vi "ziExample-PWA_SignalInput.vi"() -> ()   [LabVIEW 2009]
doc: "Control a Zurich instrument device via the LabOne Labview API. \nRequirements: Zurich Instruments UHFLI \nThis example retrives Periodic Waveform Analyzer (PWA) data from an UHFLI instrument.\n\n© Zurich Instruments AG, www.zhinst.com\\"
uses:
  <instrlib>/Zurich Instruments LabOne/Public/Data/ziTypePWAWave.ctl
  <instrlib>/Zurich Instruments LabOne/Public/Configure/ziSetValueDoubleArray.vi
  <vilib>/Analysis/2dsp.llb/Real FFT.vi
  <instrlib>/Zurich Instruments LabOne/Public/Data/ziGetEventPWAWave.vi
  <instrlib>/Zurich Instruments LabOne/Zurich Instruments LabOne.lvlib
  <vilib>/Analysis/NI_AALPro.lvlib
  <vilib>/Analysis/NI_AALBase.lvlib
panel:
  out "Error Out":errorcluster
  out "Selected Device":string
  in  "Address":string="DEV"
  in  "Bins":i32=512
  in  "stop":bool
  out "PWAWave":T1={"Timestamp (ticks)"=2149, "SampleCount"=0, "InputSelect"=0, "OscSelect"=0, "Harmonic"=0, "BinCount"=0, "Frequency (Hz)"=0.0, "PWAType"=0, "Mode"=0, "Overflow"=0, "Commensurable"=0, "BinPhase"=[], "X"=[], "Y"=[], "countBin"=[]} {"Frequency (Hz)" format="%#_6p"}
  out "FFT / Harmonics":dbl[](graph)
  out "Waveform":cluster{dbl[], dbl[]}(graph)
  out "Counts per Bin":cluster{dbl[], u32[]}(graph)
  # "ziExample-PWA.vi\nRequirements: UHFLI\nsee block diagram for VI description"
  # "Tested Devices:\n- UHFLI"
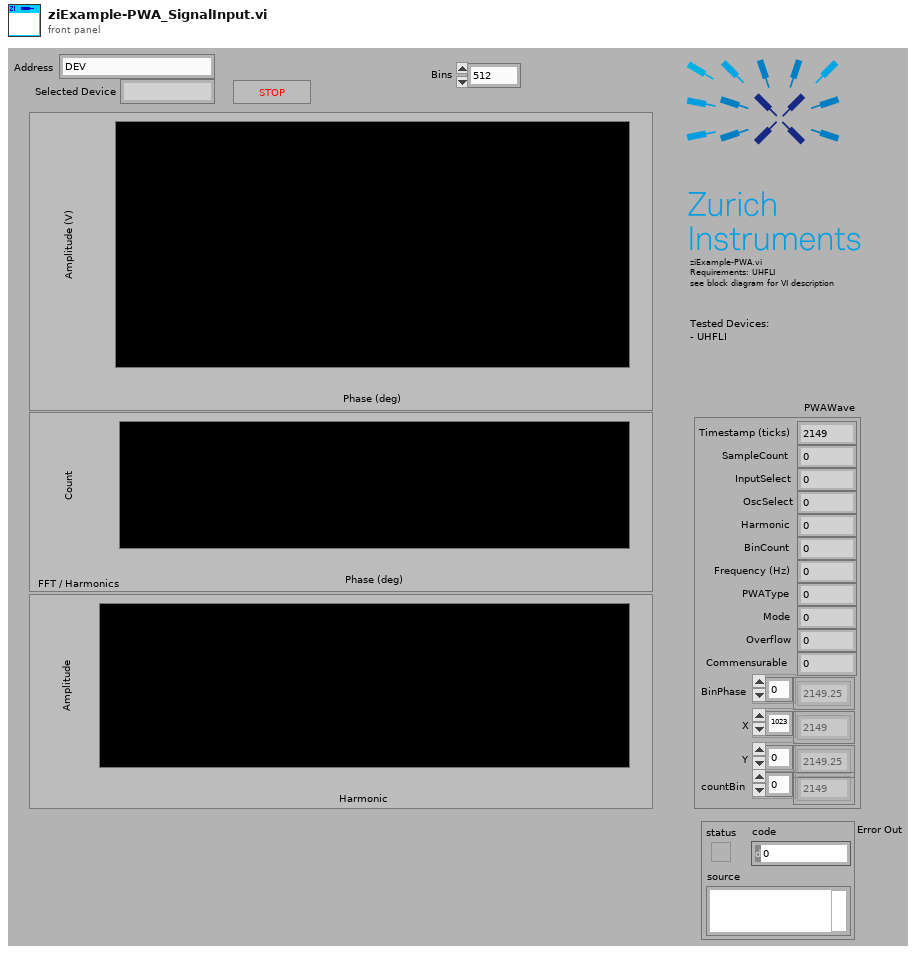
[diagram p1: front panel]
types:
  T1 = typedef "Zurich Instruments LabOne.lvlib/ziTypePWAWave.ctl" = cluster{"Timestamp (ticks)":u64, "SampleCount":u64, "InputSelect":i32, "OscSelect":i32, "Harmonic":i32, "BinCount":i32, "Frequency (Hz)":dbl, "PWAType":u8, "Mode":u8, "Overflow":u8, "Commensurable":u8, "BinPhase":dbl[], "X":dbl[], "Y":dbl[], "countBin":u32[]}
  T2 = typedef "Zurich Instruments LabOne.lvlib/ziTypeHandle.ctl" = cluster{"handleValid":bool, "Conn":u64, "Path Prefix":string, "Handle":u64, "Connected":bool, "Clockbase(s)":dbl}
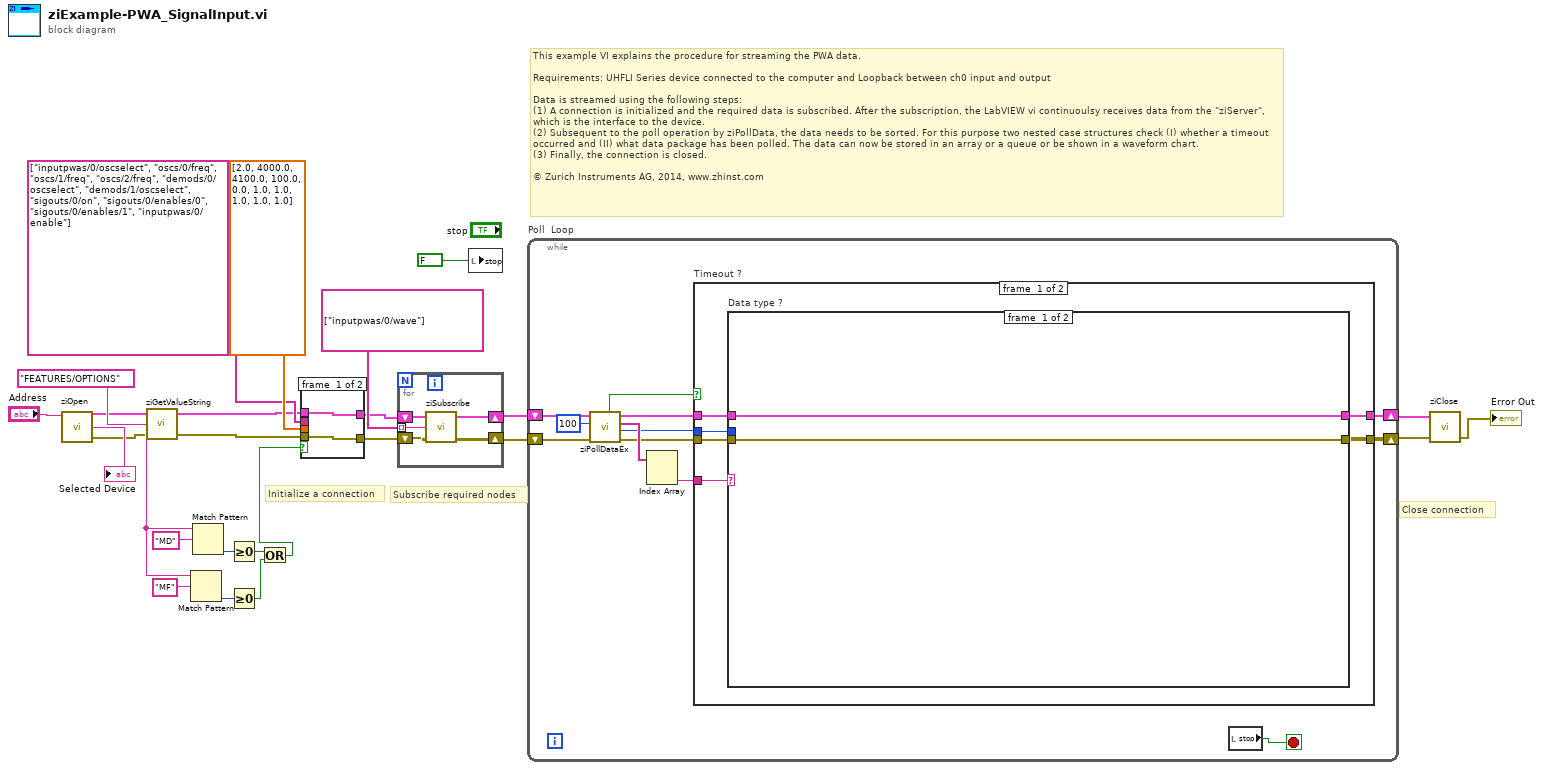
[diagram p0: block diagram]
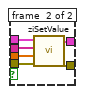
[diagram p2: hidden frame]
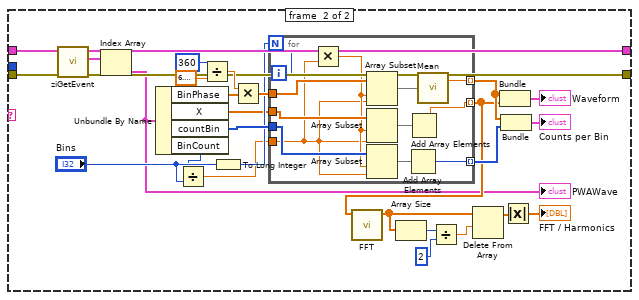
[diagram p3: hidden frame]
diagram:
  # "Close connection"
  # "Initialize a connection"
  # "Subscribe required nodes"
  # "This example VI explains the procedure for streaming the PWA data.\n\nRequirements: UHFLI Series device connected to the computer and Loopback between ch0 input and output\n\nData is streamed using the following steps:\n(1) A connection is initialized and the required data is subscribed. After the subscription, the LabVIEW vi continuoulsy receives data from the \"ziServer\", which is the interface to the device. \n(2) Subsequent to the poll operation by ziPollData, the data needs to be sorted. For this purpose two nested case structures check (I) whether a timeout occurred and (II) what data package has been polled. The data can now be stored in an array or a queue or be shown in a waveform chart. \n(3) Finally, the connection is closed. \n\n© Zurich Instruments AG, 2014, www.zhinst.com"
  n1 = call <instrlib>:"ziOpen.vi"("Address"="Address") -> ("Error Out"=w5:errorcluster, "Selected Device"=→"Selected Device":string, "HandleOut"=w2:T2)  [unwired: 1 in, 2 out]
  n2 = call <instrlib>:"ziGetValueString.vi"("error in"=w5, "Path"="FEATURES/OPTIONS", "Handle In"=w2) -> ("error out"=w4:errorcluster, "Value"=w10:string, "Handle Out"=w3:T2)
  n3 = Match Pattern(string=w10, regular expression="MF") -> (offset past match=w8:i32)  [unwired: 1 in, 3 out]
  n4 = Match Pattern(string=w10, regular expression="MD") -> (offset past match=w11:i32)  [unwired: 1 in, 3 out]
  n5 = Greater Or Equal To 0?(x=w11) -> (x >= 0?=w7:bool)
  n6 = Greater Or Equal To 0?(x=w8) -> (x >= 0?=w6:bool)
  n7 = Or(x=w7, y=w6) -> (x .or. y?=w1:bool)
  n8 = case shown="True" w1 {
    tunnel: [w28 w34] -> w18
    tunnel: [w27 w33] -> w17
    tunnel: dbl[] [2.0, 4000.0, 4100.0, 100.0, 0.0, 1.0, 1.0, 1.0, 1.0, 1.0] ("abs(x)") -> [_ w32]
    tunnel: string[] ["inputpwas/0/oscselect", "oscs/0/freq", "oscs/1/freq", "oscs/2/freq", "demods/0/oscselect", "demods/1/oscselect", "sigouts/0/on", "sigouts/0/enables/0", "sigouts/0/enables/1", "inputpwas/0/enable"] -> [_ w31]
    tunnel: w4 -> [w27 w30]
    tunnel: w3 -> [w28 w29]
    frame #0 {
    }
    frame #1 {
      n9 = call-poly <instrlib>:"ziSetValue.vi"("Error In"=w30, "Values"=w32, "Paths"=w31, "Handle In"=w29) -> ("Error Out"=w33:errorcluster, "Handle Out"=w34:T2)  [unwired: 1 in]
    }
  }
  n10 = for {
    shift-right: [w39] -> w22
    shift-left: w18 -> [w37]
    shift-right: [w38] -> w21
    shift-left: w17 -> [w36]
    tunnel: string[] ["inputpwas/0/wave"] -> [w35] mode=indexing
    n11 = call <instrlib>:"ziSubscribe.vi"("error in"=w36, "Path ()"=w35, "Handle In"=w37) -> ("error out"=w38:errorcluster, "Handle Out"=w39:T2)  [unwired: 1 in]
  }
  n12 = local write "stop"(FALSE ("Record")) -> ()
  n13 = while "Poll  Loop" {
    shift-right: [w42] -> w23
    shift-left: w22 -> [w51]
    shift-right: [w40] -> w24
    shift-left: w21 -> [w50]
    stop <- w48 stop-if-true
    n14 = call <instrlib>:"ziPollDataEx.vi"("error in"=w50, "Timeout ms (50)"=100 ("TimeOut ms (50)"), "Handle In"=w51) -> ("error out"=w41:errorcluster, "Timestamp (ticks)"=w44:u64, "PathArray"=w46:string[], "Handle Out"=w43:T2, "Timed Out"=w47:bool)  [unwired: 1 in, 3 out]
    n15 = Index Array(array=w46) -> (element #2=w45:string)  [unwired: 2 in, 1 out]
    n16 = case "Timeout ?" shown="False" w47 {
      tunnel: w45 -> [w57 _]
      tunnel: w44 -> [w56 _]
      tunnel: w43 -> [w55 w101]
      tunnel: [w54 w101] -> w42
      tunnel: w41 -> [w53 w100]
      tunnel: [w52 w100] -> w40
      frame #0 {
        n17 = case "Data type ?" shown="\"INPUTPWAS\"" w57 {
          tunnel: w56 -> [_ _]
          tunnel: w55 -> [w59 w87]
          tunnel: [w59 w86] -> w54
          tunnel: w53 -> [w58 w74]
          tunnel: [w58 w73] -> w52
          frame #0 {
          }
          frame #1 {
            n18 = call-poly <instrlib>:"ziGetEvent.vi"("Error In"=w74, "Handle In"=w87) -> ("Error Out"=w73:errorcluster, "PWAWaves Out"=w72:T1[], "Handle Out"=w86:T2)  [unwired: 7 in]
            n19 = Index Array(array=w72) -> (element=w63:T1)  [unwired: 1 in]
            "PWAWave" <- w63
            n20 = Unbundle By Name(w63) -> ("BinPhase"=w61:dbl[], "X"=w62:dbl[], "countBin"=w85:u32[], "BinCount"=w60:i32)
            n21 = Divide(x=w60, y="Bins") -> (x/y=w65:dbl)
            n22 = Divide(x=360, y=6.283185307179586) -> (x/y=w82:dbl)
            n23 = To Long Integer(number="Bins") -> (32bit integer=w67:i32)
            n24 = Multiply(x=w82, y=w61) -> (x*y=w81:dbl[])
            n25 = for {
              N: w67 -> [_]
              tunnel: w85 -> [w97]
              tunnel: w81 -> [w99]
              tunnel: w62 -> [w93]
              tunnel: w65 -> [w91]
              tunnel: [w89] -> w71 mode=indexing
              tunnel: [w94] -> w70 mode=indexing
              tunnel: [w88] -> w64 mode=indexing
              i -> [w98]
              n26 = Multiply(x=w98, y=w91) -> (x*y=w92:dbl)
              n27 = Array Subset(array=w99, index=w92, length=w91) -> (w95:dbl[])
              n28 = Array Subset(array=w93, index=w92, length=w91) -> (w90:dbl[])
              n29 = Array Subset(array=w97, index=w92, length=w91) -> (w96:u32[])
              n30 = Add Array Elements(numeric array=w96) -> (sum=w89:u32)
              n31 = Add Array Elements(numeric array=w90) -> (sum=w88:dbl)
              n32 = call <vilib>:"Mean.vi"("X"=w95) -> ("mean"=w94:dbl)  [unwired: 1 out]
            }
            n33 = call-poly <vilib>:"FFT.vi"("X"=w64) -> ("FFT {X}"=w78:cdb[])  [unwired: 9 in, 1 out]
            n34 = Array Size(array=w78) -> (size(s)=w77:i32)
            n35 = Divide(x=w77, y=2) -> (x/y=w75:dbl)
            n36 = Delete From Array(array=w78, length=w75) -> (array with subset deleted=w79:cdb[])  [unwired: 1 in, 1 out]
            n37 = Bundle(w70, w64) -> (→"Waveform":cluster{dbl[], dbl[]})  [unwired: 1 in]
            n38 = Bundle(w70, w71) -> (→"Counts per Bin":cluster{dbl[], u32[]})  [unwired: 1 in]
            n39 = Absolute Value(x=w79) -> (abs(x)=→"FFT / Harmonics":dbl[])
          }
        }
      }
      frame #1 {
        # "Timeout, no action."
      }
    }
    n40 = local read "stop"() -> (w48:bool)
  }
  n41 = call <instrlib>:"ziClose.vi"("Error In"=w24, "Handle In"=w23) -> ("Error Out"=→"Error Out":errorcluster)  [unwired: 3 out]
